vi "Test Pass.vi"(11 "Test Case In":refnum<class "API Pass Output.lvclass">) -> (0 "error out":errorcluster, 3 "Test Case Out":refnum<class "API Pass Output.lvclass">)   [LabVIEW 2020, in "API Pass Output.lvclass"]
uses:
  API Pass Output.lvclass
  API Pass Output.lvclass/API Pass Output.ctl
  4993e8ee-a06a-463a-9684-69129f64d5ce.vi
  source/User Interface/Execution API/Execution API.lvclass
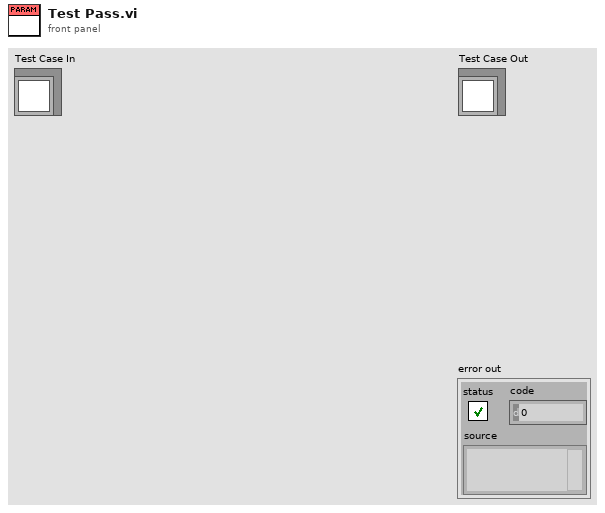
[diagram p1: front panel]
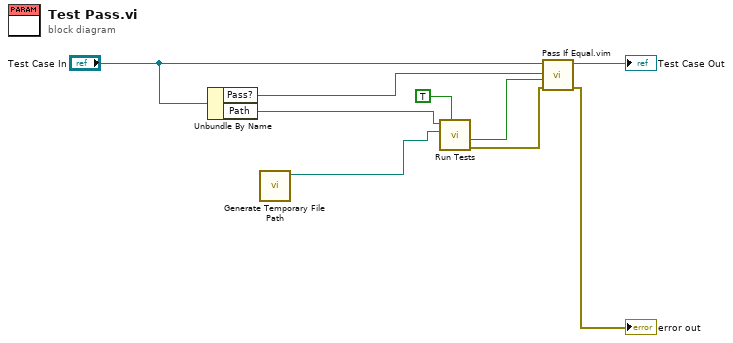
[diagram p0: block diagram]
diagram:
  n1 = Unbundle By Name("Test Case In") -> ("Pass?"=w6:bool, "Path"=w5:path)
  n2 = call <vilib>:"Generate Temporary File Path.vi"() -> ("Unique Temporary File Path"=w4:path)  [unwired: 10 in, 1 out]
  n3 = call "Run Tests.vi"("Run Tests In Parallel? (T)"=TRUE, "Report Output path"=w4, "Project, Library, or Test Class Path"=w5) -> ("error out"=w2:errorcluster, "All Passed?"=w3:bool)  [unwired: 6 in, 1 out]
  n4 = call "Pass If Equal.vim"("error in (no error)"=w2, "Actual"=w3, "Expected"=w6, "LUnit Test Case In"="Test Case In") -> ("error out"=→"error out":errorcluster, "LUnit Test Case Out"=→"Test Case Out":refnum<class "API Pass Output.lvclass">)  [unwired: 6 in]
